vi "Plan Line, Constant Velocity.vi"(6 "Side":T3=enum."right", 8 "Joints":dbl[](array[numeric]), 10 "queue":refnum<queue>, 11 "Goal":T1) -> (1 "Q size":i32)   [LabVIEW 2013]
uses:
  ROS/Code/SubVIs/BaxterSide.ctl
  Goal.ctl
  <vilib>/Analysis/Matrix/Datatypes/RealMatrix.ctl
  Fwd Kenimatics - array.vi
  Baxter Examples/Arm Globals.vi
  <vilib>/Analysis/Matrix/NI_Matrix.lvlib
panel:
  in  "Stop":bool
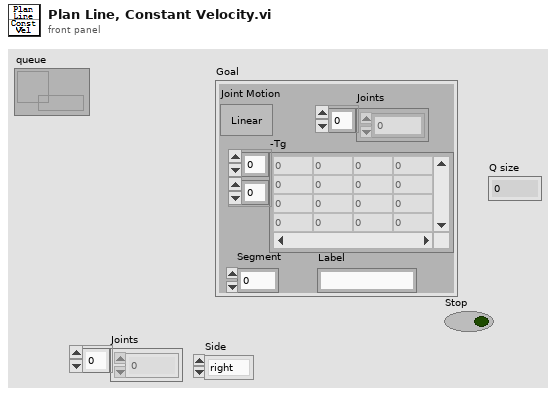
[diagram p1: front panel]
types:
  T1 = typedef "Goal.ctl" = cluster{"Segment":dbl, "-Tg":T2, "Joints":dbl[], "Label":string, "Joint Motion":bool}
  T2 = typedef "NI_Matrix.lvlib/RealMatrix.ctl" = dbl[][]
  T3 = typedef "BaxterSide.ctl" = enum16{"left", "right"}
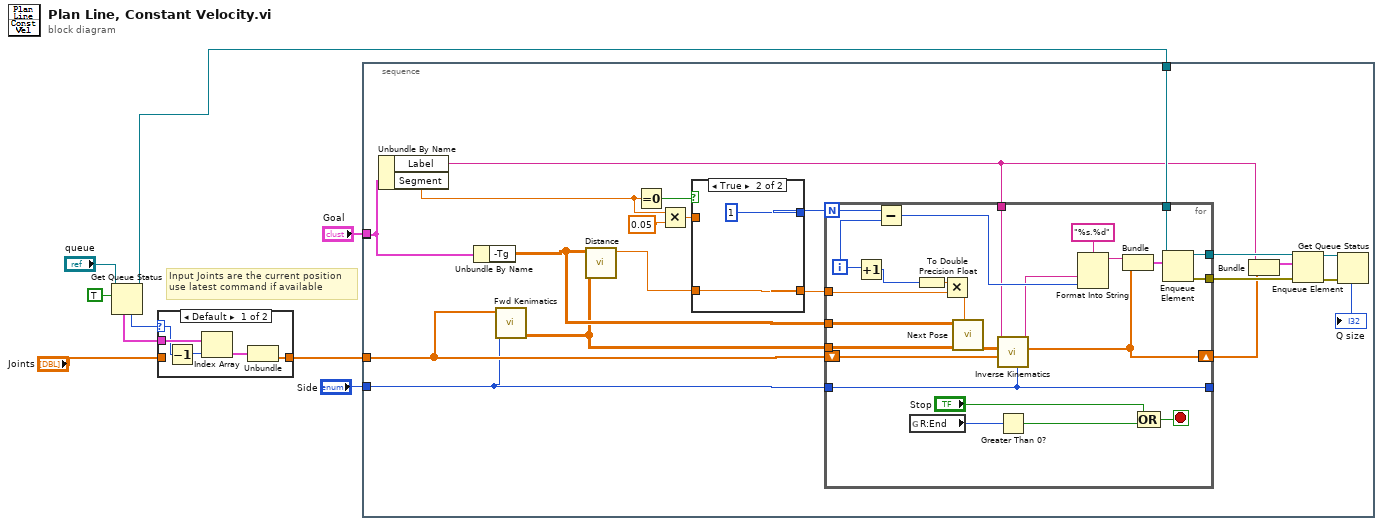
[diagram p0: block diagram]
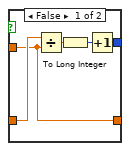
[diagram p3: hidden frame]
diagram:
  # "Input Joints are the current position\nuse latest command if available"
  n1 = Get Queue Status(queue="queue", return elements? (F)=TRUE) -> (queue out=w2:refnum<queue>, # elements in queue=w7:i32, elements=w5:cluster{string, "Joints":dbl[]}[])  [unwired: 1 in, 5 out]
  n2 = case shown="Default" w7 {
    selector: w7 -> [w13 _]
    tunnel: w5 -> [w14 _]
    tunnel: [w10 w15] -> w4
    tunnel: "Joints" -> [_ w15]
    frame Default {
      n3 = Decrement(x=w13) -> (x-1=w12:i32)
      n4 = Index Array(array=w14, index=w12) -> (element=w11:cluster{string, "Joints":dbl[]})
      n5 = Unbundle(w11) -> ("Joints"=w10:dbl[])  [unwired: 1 out]
    }
    frame 0 {
    }
  }
  n6 = stacked-sequence {
    tunnel: w2 -> [w35]
    tunnel: "Side" -> [w17]
    tunnel: w4 -> [w21]
    tunnel: [w16] -> _
    tunnel: "Goal" -> [w16]
    frame #0 {
      n7 = Unbundle By Name(w16) -> ("Label"=w28:string, "Segment"=w22:dbl)
      n8 = Unbundle By Name(w16) -> ("-Tg"=w19:T2)
      n9 = call-poly "Fwd Kenimatics.vi"("Side"=w17, "Joints"=w21) -> ("Matrix"=w18:T2)  [unwired: 8 in, 1 out]
      n10 = call "Distance.vi"("Pose 2"=w18, "Pose 1"=w19) -> ("Distance"=w20:dbl)  [unwired: 9 in]
      n11 = Equal To 0?(x=w22) -> (x = 0?=w32:bool)
      n12 = Multiply(x=w22, y=0.05) -> (x*y=w23:dbl)
      n13 = case shown="True" w32 {
        tunnel: w20 -> [w66 w68]
        tunnel: [w63 w68] -> w36
        tunnel: [w62 1] -> w34
        tunnel: w23 -> [w63 _]
        frame False {
          n14 = Divide(x=w66, y=w63) -> (x/y=w64:dbl)
          n15 = To Long Integer(number=w64) -> (32bit integer=w65:i32)
          n16 = Increment(x=w65) -> (x+1=w62:i32)
        }
        frame True {
        }
      }
      n17 = for {
        N: w34 -> [w52]
        tunnel: w19 -> [w61]
        tunnel: w18 -> [w60]
        tunnel: w36 -> [w54]
        shift-right: [w47] -> w27
        shift-left: w21 -> [w56]
        tunnel: w35 -> [w59]
        tunnel: [w58] -> w31
        tunnel: [w57] -> w30
        tunnel: w17 -> [w40]
        tunnel: [w40] -> _
        tunnel: w28 -> [w39]
        i -> [w51]
        stop <- w45 stop-if-true
        n18 = Increment(x=w51) -> (x+1=w55:i32)
        n19 = Subtract(x=w52, y=w51) -> (x-y=w49:i32)
        n20 = global read "Arm Globals.vi" "R:End"() -> (w44:i32)
        n21 = To Double Precision Float(number=w55) -> (double precision float=w53:dbl)
        n22 = Multiply(x=w53, y=w54) -> (x*y=w43:dbl)
        n23 = call "Next Pose.vi"("Step"=w43, "Last Pose"=w60, "Goal"=w61) -> ("Pose"=w42:T2)  [unwired: 7 in, 1 out]
        n24 = call "Inverse Kinematics.vi"("Side"=w40, "Start"=w56, "Goal-matrix"=w42, "Label"=w39) -> ("J"=w47:dbl[], "Label"=w38:string)  [unwired: 4 in, 2 out]
        n25 = Greater Than 0?(x=w44) -> (x > 0?=w37:bool)
        n26 = Format Into String(format string="%s.%d", w38, w49) -> (resulting string=w48:string)  [unwired: 2 in, 1 out]
        n27 = Bundle(w48, "J"=w47) -> (w46:cluster{string, "J":dbl[]})  [unwired: 1 in]
        n28 = Compound Arithmetic op=OR("Stop", w37) -> (w45:bool)
        n29 = Enqueue Element(queue=w59, element=w46) -> (queue out=w58:refnum<queue>, error out=w57:errorcluster)  [unwired: 2 in, 1 out]
      }
      n30 = Bundle("Label"=w28, "Joints"=w27) -> (w29:cluster{"Label":string, "Joints":dbl[]})  [unwired: 1 in]
      n31 = Enqueue Element(queue=w31, element=w29, error in (no error)=w30) -> (queue out=w26:refnum<queue>, error out=w25:errorcluster)  [unwired: 1 in, 1 out]
      n32 = Get Queue Status(queue=w26, error in (no error)=w25) -> (# elements in queue=→"Q size":i32)  [unwired: 1 in, 7 out]
    }
  }
